vi "S&E Message Output.vi"(1 "All analog ch data":dbl[](array[numeric]), 2 "All digital Ch data":T2[](array[typedef]), 5 "Type(File Hist)":T1, 7 "E&S Message":T3, 9 "error in (no error)":errorcluster, 12 "Time format(%T)":string="%T", 13 "Delimiter(;)":string=";") -> (6 "String(File)":string, 8 "Array of strings":string[](array[string]), 10 "error out":errorcluster)   [LabVIEW 2011]
uses:
  emi Lib/System 01/0 - General/S&E reporting/Private/_emi_ S&E Message.ctl
  emi Lib/System 01/0 - General/S&E reporting/Private/_emi_ S&E Message type.ctl
  Measurments Handling/Status Digitalish.ctl
  String outpyt type.ctl
  reate/S&E Analog Alarm type.ctl
  GUI/Status Indikator Helper.ctl
  reate/S&E Event Type.ctl
  reate/S&E Event source.ctl
  reate/S&E Digital Alarm Type.ctl
  reate/S&E Anotationtype.ctl
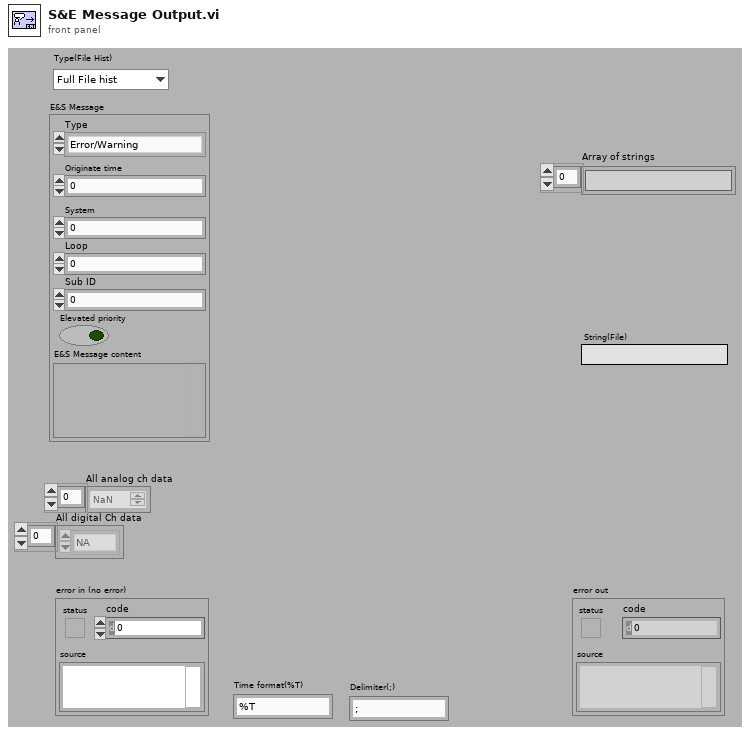
[diagram p1: front panel]
types:
  T1 = typedef "String outpyt type.ctl" = enum16{"Full File hist", "Simple File hist", "Displ Hist one type", "Displ Hist mult types", "Displ Stat one type", "Displ Stat Mult type"}
  T2 = typedef "Status Digitalish.ctl" = enum16{"NA", "False", "True"}
  T3 = typedef "_emi_ S&E Message.ctl" = cluster{"Type":T4, "Originate time":dbl, "System":u8, "Loop":u16, "Sub ID":u16, "Elevated priority":bool, "E&S Message content":variant}
  T4 = typedef "_emi_ S&E Message type.ctl" = enum16{"Error/Warning", "Note", "Debug", "Event", "Alarm Analog", "Alarm Digital", "Annotation"}
  T5 = typedef "S&E Analog Alarm type.ctl" = cluster{"Alarm":bool, "State":T6, "Value":dbl, "Source name":string}
  T6 = typedef "Status Indikator Helper.ctl" = enum16{"Norm", "L", "H", "LL", "HH", "Value", "Technical"}
  T7 = typedef "S&E Event Type.ctl" = cluster{"Event Source":T8, "Source Info":string, "Event Description":string}
  T8 = typedef "S&E Event source.ctl" = enum16{"User", "Instrument", "Application", "Windows"}
  T9 = typedef "S&E Digital Alarm Type.ctl" = cluster{"Alarm":bool, "Enum":T6, "Value":T2, "Source name":string, "Status text":string}
  T10 = typedef "S&E Anotationtype.ctl" = cluster{"User":string, "Annotation":string}
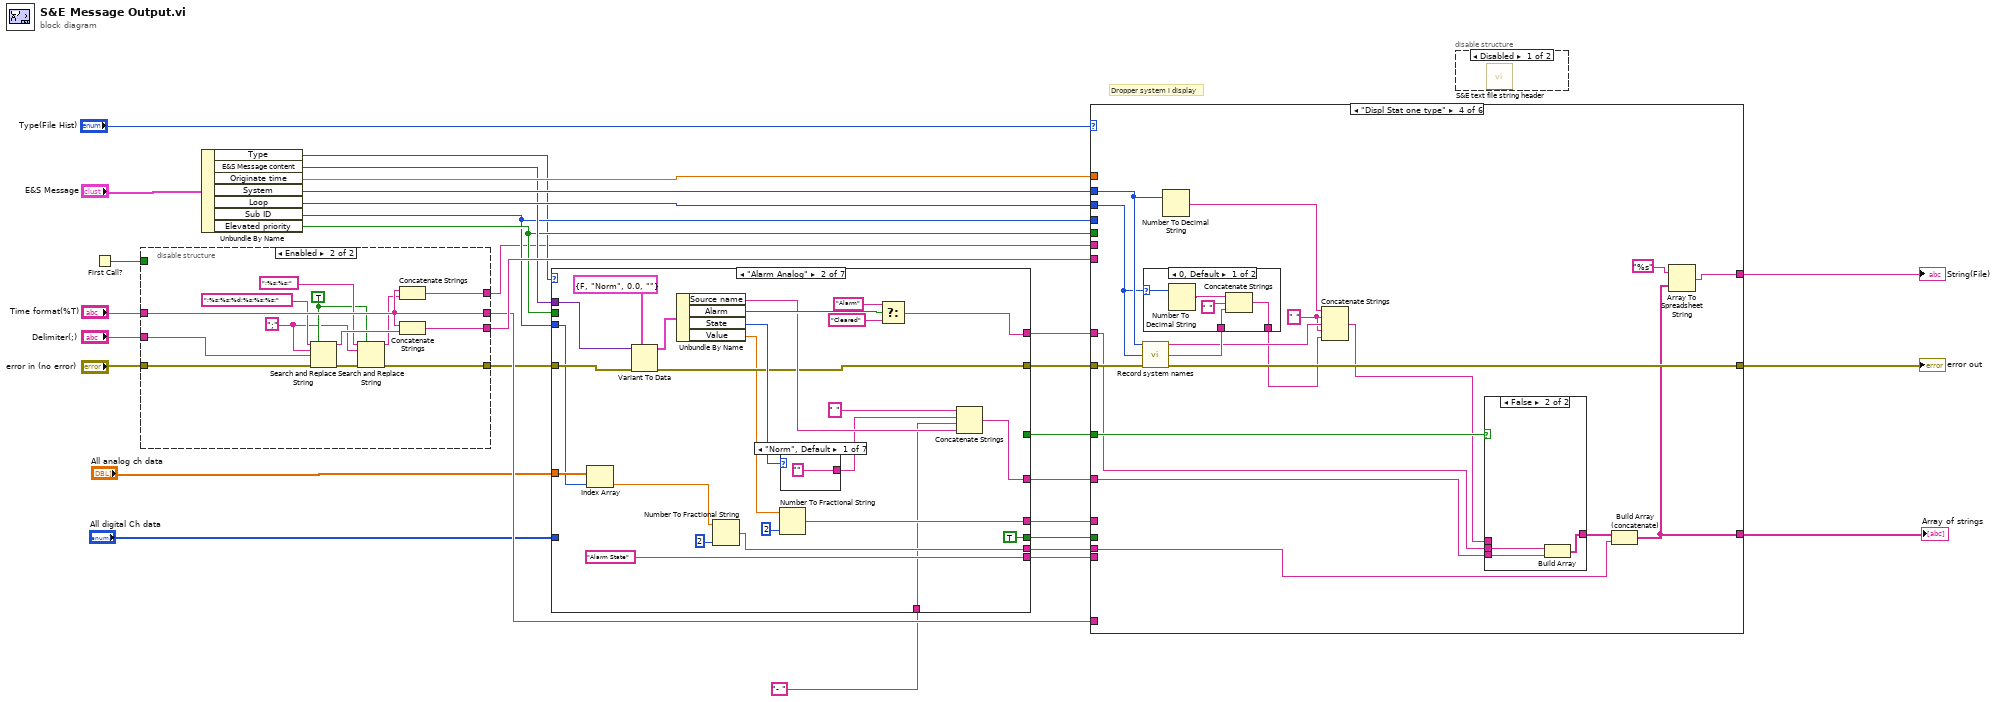
[diagram p0: block diagram]
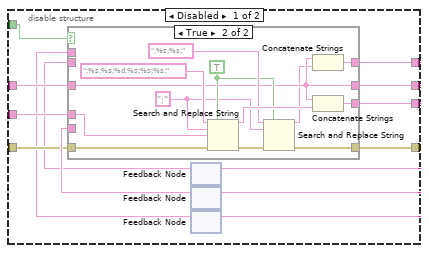
[diagram p2: hidden frame]
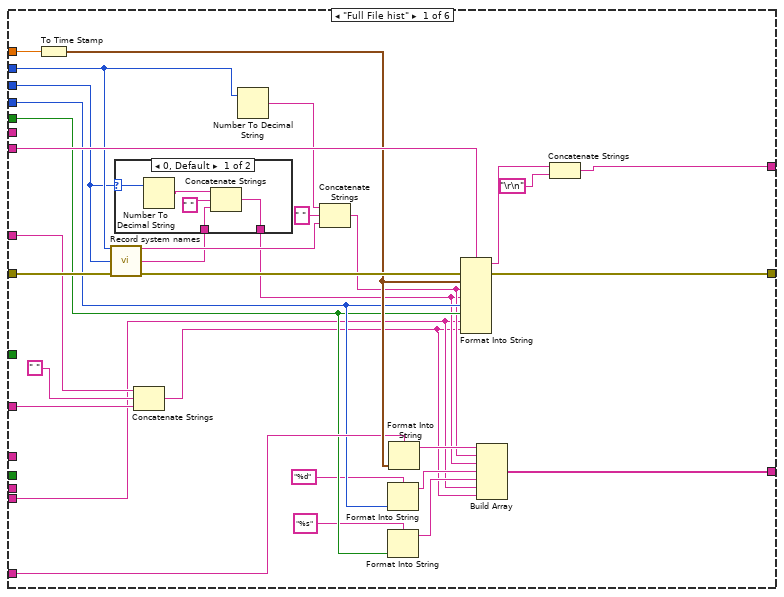
[diagram p5: hidden frame]
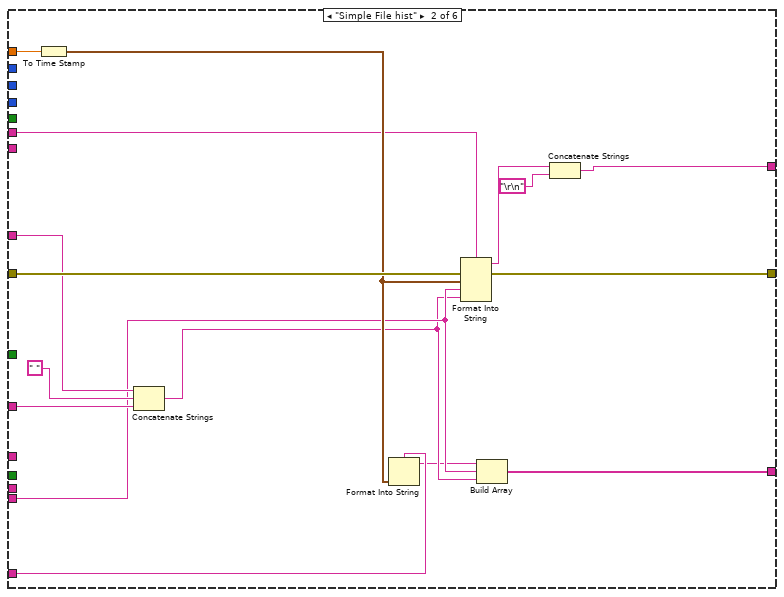
[diagram p7: hidden frame]
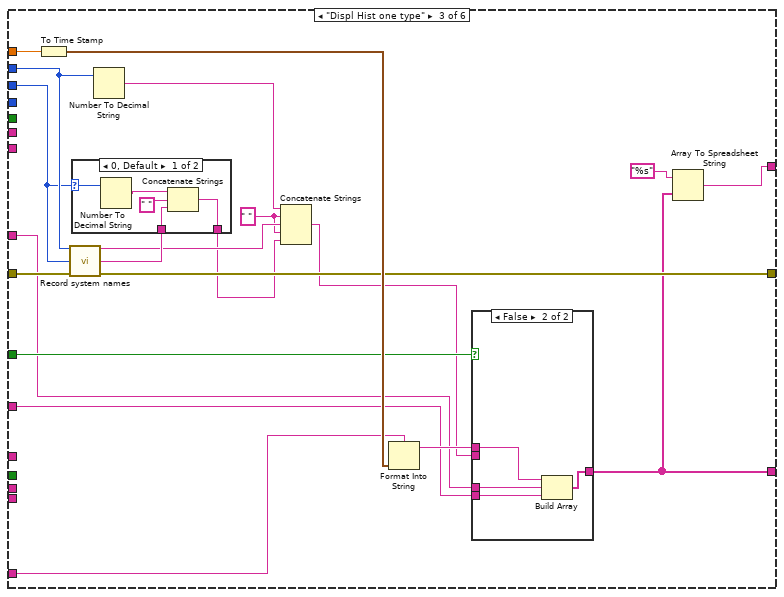
[diagram p8: hidden frame]
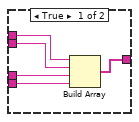
[diagram p9: hidden frame]
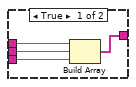
[diagram p11: hidden frame]
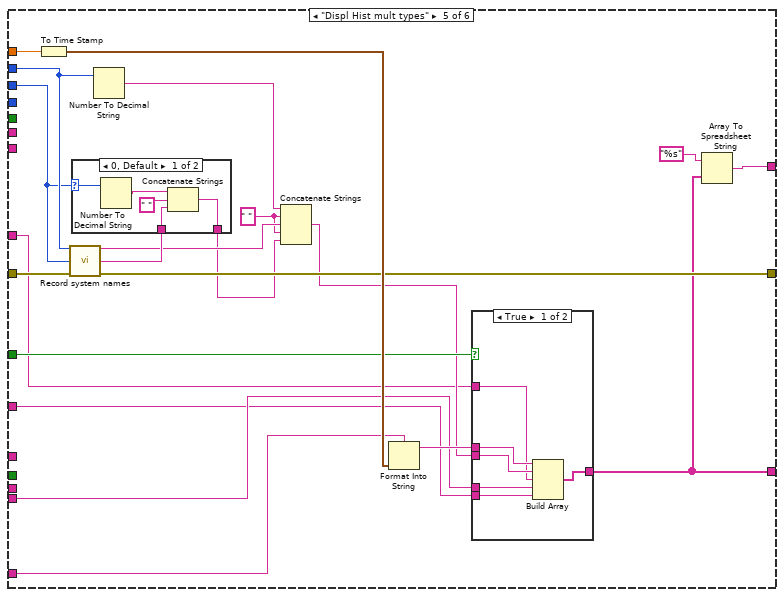
[diagram p13: hidden frame]
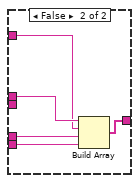
[diagram p14: hidden frame]
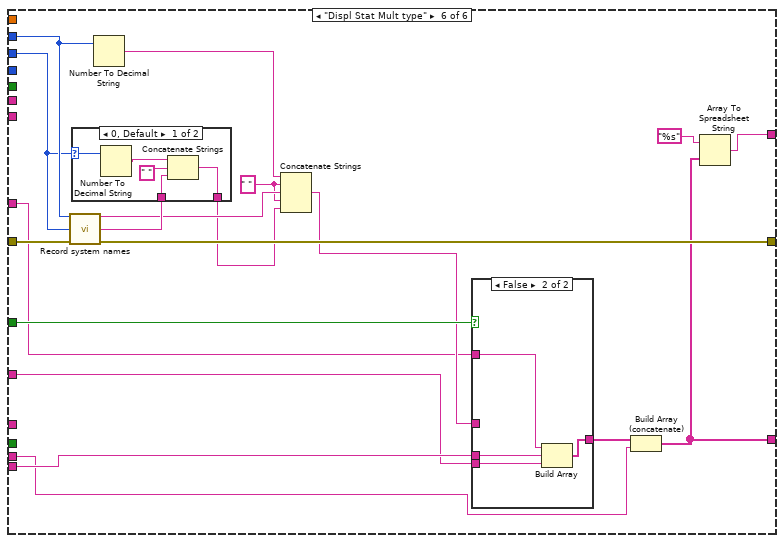
[diagram p16: hidden frame]
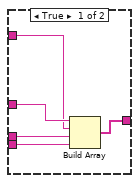
[diagram p17: hidden frame]
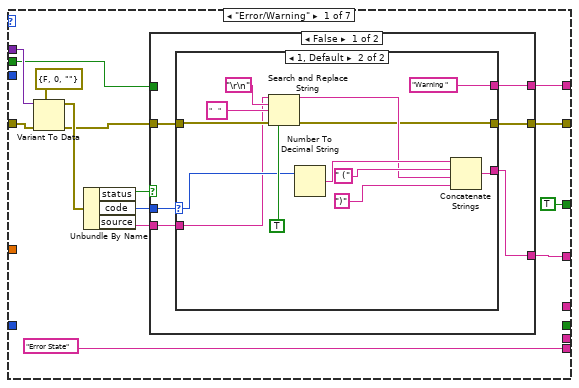
[diagram p19: hidden frame]
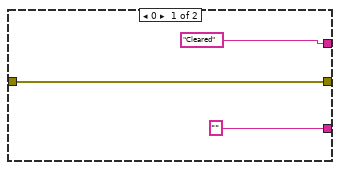
[diagram p20: hidden frame]
diagram:
  # "Dropper system i display"
  n1 = First Call?() -> (First Call?: T/F=w31:bool)
  n2 = disable-structure shown="Enabled" {
    disable-tunnel: w31 -> [w41 _]
    disable-tunnel: "Delimiter(;)" -> [w40 w72]
    disable-tunnel: "Time format(%T)" -> [w39 w69]
    disable-tunnel: "error in (no error)" -> [w38 w71]
    disable-tunnel: [w37 w70] -> w23
    disable-tunnel: [w35 w69] -> w20
    disable-tunnel: [w34 w68] -> w18
    disable-tunnel: [w32 w67] -> w2
    frame Disabled {
      n3 = feedback #1() -> (w33:string)  [unwired: 1 in]
      n4 = feedback #2() -> (w42:string)  [unwired: 1 in]
      n5 = feedback #3() -> (w36:string)  [unwired: 1 in]
      n6 = case shown="True" w41 {
        tunnel: [w46 w59] -> w37
        tunnel: w39 -> [_ w49]
        tunnel: w40 -> [_ w56]
        tunnel: w42 -> [w46 _]
        tunnel: [w45 w53] -> w34
        tunnel: w38 -> [w45 w55]
        tunnel: [w44 w49] -> w35
        tunnel: w36 -> [w44 _]
        tunnel: [w43 w47] -> w32
        tunnel: w33 -> [w43 _]
        frame False {
        }
        frame True {
          w51 = TRUE ("replace all? (F)")
          w50 = ";" ("search string")
          n7 = Search and Replace String(replace all?=w51, input string=";%s;%s;%d;%s;%s;%s;" ("format string"), search string=w50, replace string=w56, error in=w55) -> (result string=w58:string, error out=w54:errorcluster)  [unwired: 3 in, 2 out]
          n8 = Search and Replace String(replace all?=w51, input string=";%s;%s;" ("format string"), search string=w50, error in=w54) -> (result string=w48:string, error out=w53:errorcluster)  [unwired: 4 in, 2 out]
          n9 = Concatenate Strings(w49, w48) -> (w47:string)
          n10 = Concatenate Strings(w49, w58) -> (w59:string)
        }
      }
      n11 = feedback-in #1(w32) -> ()
      n12 = feedback-in #2(w37) -> ()
      n13 = feedback-in #3(w35) -> ()
    }
    frame Enabled {
      w62 = TRUE ("replace all? (F)")
      w61 = ";" ("search string")
      n14 = Search and Replace String(replace all?=w62, input string=";%s;%s;%d;%s;%s;%s;" ("format string"), search string=w61, replace string=w72, error in=w71) -> (result string=w66:string, error out=w64:errorcluster)  [unwired: 3 in, 2 out]
      n15 = Search and Replace String(replace all?=w62, input string=";%s;%s;" ("format string"), search string=w61, error in=w64) -> (result string=w60:string, error out=w68:errorcluster)  [unwired: 4 in, 2 out]
      n16 = Concatenate Strings(w69, w60) -> (w67:string)
      n17 = Concatenate Strings(w69, w66) -> (w70:string)
    }
  }
  n18 = Unbundle By Name("E&S Message") -> ("Type"=w9:T4, "E&S Message content"=w17:variant, "Originate time"=w26:dbl, "System"=w22:u8, "Loop"=w21:u16, "Sub ID"=w13:u16, "Elevated priority"=w16:bool)
  n19 = case shown="\"Alarm Analog\"" w9 {
    tunnel: [w75 w132 w160 w184 w207 w214 w222] -> w19
    tunnel: w18 -> [w83 w143 w164 w194 w210 w218 w225]
    tunnel: w17 -> [w82 w142 w163 w193 w209 w217 w224]
    tunnel: w16 -> [w79 _ _ _ _ _ _]
    tunnel: ["Error State" ("Time format(%T)") "Alarm State" ("Time format(%T)") "Event" ("Time format(%T)") "Alarm State" ("Time format(%T)") "User annotation" ("Time format(%T)") "Info" ("Time format(%T)") "Debug Message" ("Time format(%T)")] -> w12
    tunnel: [w76 w137 w157 w188 w204 _ _] -> w10
    tunnel: [w74 w133 w161 w185 w206 w215 w223] -> w11
    tunnel: [_ w130 _ w172 _ _ _] -> w6
    tunnel: "All analog ch data" -> [_ w129 _ _ _ _ _]
    tunnel: "All digital Ch data" -> [_ _ _ w181 _ _ _]
    tunnel: w13 -> [_ w128 _ w183 _ _ _]
    tunnel: [_ w126 _ w177 _ _ _] -> w5
    tunnel: [TRUE _ _ _ _ TRUE TRUE] -> w4
    tunnel: [_ TRUE _ TRUE _ _ _] -> w3
    tunnel: "- " ("string") -> [_ w122 w154 w179 _ _ _]
    frame "Error/Warning" {
      n20 = Variant To Data(error in=w83, type=errorcluster {"status"=FALSE, "code"=0, "source"=""} ("error in (no error)"), Variant=w82) -> (data=w84:errorcluster, error out=w80:errorcluster)
      n21 = Unbundle By Name(w84) -> ("status"=w81:bool, "code"=w78:i32, "source"=w77:string)
      n22 = case shown="False" w81 {
        tunnel: w80 -> [w92 w113]
        tunnel: w79 -> [_ _]
        tunnel: w78 -> [w87 w117]
        tunnel: w77 -> [w88 w112]
        tunnel: [w90 "Error" ("format string")] -> w76
        tunnel: [w91 w111] -> w75
        tunnel: [w89 w109] -> w74
        frame False {
          n23 = case shown="1, Default" w87 {
            selector: w87 -> [_ w99]
            tunnel: ["" w97] -> w89
            tunnel: [w95 w100] -> w91
            tunnel: w92 -> [w95 w101]
            tunnel: w88 -> [_ w98]
            tunnel: ["Cleared" ("format string") "Warning " ("format string")] -> w90
            frame 0 {
            }
            frame 1, Default {
              n24 = Search and Replace String(replace all?=TRUE ("replace all? (F)"), input string=w98, search string="\r\n", replace string="   " ("format string"), error in=w101) -> (result string=w104:string, error out=w100:errorcluster)  [unwired: 3 in, 2 out]
              n25 = Number To Decimal String(number=w99) -> (decimal integer string=w108:string)  [unwired: 1 in]
              n26 = Concatenate Strings(w108, " (" ("string"), w104, ")" ("string")) -> (w97:string)
            }
          }
        }
        frame True {
          n27 = Number To Decimal String(number=w117) -> (decimal integer string=w121:string)  [unwired: 1 in]
          n28 = Search and Replace String(replace all?=TRUE ("replace all? (F)"), input string=w112, search string="\r\n", replace string="   " ("format string"), error in=w113) -> (result string=w110:string, error out=w111:errorcluster)  [unwired: 3 in, 2 out]
          n29 = Concatenate Strings(w121, " (" ("string"), w110, ")" ("string")) -> (w109:string)
        }
      }
    }
    frame "Alarm Analog" {
      n30 = Index Array(array=w129, index=w128) -> (element=w127:dbl)
      n31 = Variant To Data(error in=w143, type=T5 {"Alarm"=FALSE, "State"=enum."Norm", "Value"=0.0, "Source name"=""} ("S&E Alarm"), Variant=w142) -> (data=w145:T5, error out=w132:errorcluster)
      n32 = Unbundle By Name(w145) -> ("Source name"=w135:string, "Alarm"=w140:bool, "State"=w138:T6, "Value"=w131:dbl)
      n33 = Number To Fractional String(number=w127, precision (6)=i16 2) -> (F-format string=w126:string)  [unwired: 2 in]
      n34 = Number To Fractional String(number=w131, precision (6)=i16 2) -> (F-format string=w130:string)  [unwired: 2 in]
      n35 = case shown="\"Norm\", Default" w138 {
        tunnel: ["" ("string") "L" ("string") "H" ("string") "LL" ("string") "HH" ("string") "Tech" ("string") "Dig" ("string")] -> w134
        frame "Norm", Default {
        }
        frame "L" {
        }
        frame "H" {
        }
        frame "LL" {
        }
        frame "HH" {
        }
        frame "Technical" {
        }
        frame "Value" {
        }
      }
      n36 = Select(t="Alarm", s=w140, f="Cleared") -> (s? t:f=w137:string)
      n37 = Concatenate Strings(" " ("string"), w134, w122, w135) -> (w133:string)
    }
    frame "Event" {
      n38 = Variant To Data(error in=w164, type=T7 {"Event Source"=enum."User", "Source Info"="", "Event Description"=""} ("S&E Event"), Variant=w163) -> (data=w165:T7, error out=w160:errorcluster)
      n39 = Unbundle By Name(w165) -> ("Event Description"=w155:string, "Source Info"=w156:string, "Event Source"=w158:T8)
      n40 = case shown="\"Application\"" w158 {
        tunnel: ["User" ("string") "Win." ("string") "Inst." ("string") "App." ("string")] -> w157
        frame "User", Default {
        }
        frame "Windows" {
        }
        frame "Instrument" {
        }
        frame "Application" {
        }
      }
      n41 = Concatenate Strings(w156, " " ("string"), w155, w154) -> (w161:string)
    }
    frame "Alarm Digital" {
      n42 = Index Array(array=w181, index=w183) -> (element=w178:T2)
      n43 = Variant To Data(error in=w194, type=T9 {"Alarm"=FALSE, "Enum"=enum."Norm", "Value"=enum."NA", "Source name"="", "Status text"=""} ("S&E Alarm"), Variant=w193) -> (data=w195:T9, error out=w184:errorcluster)
      n44 = Format Into String(format string="%s", w178) -> (resulting string=w177:string)  [unwired: 2 in, 1 out]
      n45 = Unbundle By Name(w195) -> ("Source name"=w171:string, "Alarm"=w191:bool, "Enum"=w189:T6, "Value"=w174:T2, "Status text"=w173:string)
      n46 = case shown="\"L\"" w189 {
        tunnel: ["" ("string") "L" ("string") "H" ("string") "LL" ("string") "HH" ("string") "Tech" ("string") "Val" ("string")] -> w186
        frame "Norm", Default {
        }
        frame "L" {
        }
        frame "H" {
        }
        frame "LL" {
        }
        frame "HH" {
        }
        frame "Technical" {
        }
        frame "Value" {
        }
      }
      n47 = Format Into String(format string="%s(%s)", w174, w173) -> (resulting string=w172:string)  [unwired: 2 in, 1 out]
      n48 = Select(t="Alarm", s=w191, f="Cleared") -> (s? t:f=w188:string)
      n49 = Concatenate Strings(" " ("string"), w186, w179, w171) -> (w185:string)
    }
    frame "Annotation" {
      (unwired) "   " ("string")
      n50 = Variant To Data(error in=w210, type=T10 {"User"="", "Annotation"=""} ("S&E Alarm"), Variant=w209) -> (data=w211:T10, error out=w207:errorcluster)
      n51 = Unbundle By Name(w211) -> ("User"=w204:string, "Annotation"=w208:string)
      n52 = Concatenate Strings(w208) -> (w206:string)
    }
    frame "Note" {
      n53 = Variant To Data(error in=w218, type="" ("Measage Header string"), Variant=w217) -> (data=w215:string, error out=w214:errorcluster)
    }
    frame "Debug" {
      n54 = Variant To Data(error in=w225, type="" ("Measage Header string"), Variant=w224) -> (data=w223:string, error out=w222:errorcluster)
    }
  }
  n55 = case shown="\"Displ Stat one type\"" "Type(File Hist)" {
    tunnel: [w231 w270 w280 w317 w347 w387] -> w30
    tunnel: w26 -> [w256 w278 w299 _ w366 _]
    tunnel: [w255 w277 w289 w326 w355 w395] -> w24
    tunnel: w23 -> [w254 _ _ _ _ _]
    tunnel: w22 -> [w249 _ w297 w331 w364 w401]
    tunnel: w21 -> [w248 _ w296 w330 w363 w400]
    tunnel: w20 -> [w242 w272 w292 _ w359 _]
    tunnel: w19 -> [w246 w276 w294 w328 w361 w398]
    tunnel: w16 -> [w240 _ _ _ _ _]
    tunnel: w13 -> [w241 _ _ _ _ _]
    tunnel: w12 -> [w228 w266 _ _ w357 w397]
    tunnel: w11 -> [w245 w275 w290 w327 w356 w396]
    tunnel: w10 -> [w244 w274 w283 w320 w349 w389]
    tunnel: [w232 w271 w282 w316 w346 w385] -> w7
    tunnel: w6 -> [_ _ _ _ _ _]
    tunnel: w5 -> [_ _ _ w315 _ w384]
    tunnel: w4 -> [_ _ w288 w325 w354 w394]
    tunnel: w3 -> [_ _ _ _ _ _]
    tunnel: w2 -> [_ w267 _ _ _ _]
    frame "Full File hist" {
      n56 = To Time Stamp(1:w256) -> (0:w243:timestamp)
      n57 = call "Record system names.vi"("System(0)"=w249, "Loop(0)"=w248, "error in (no error)"=w246) -> ("System navn"=w250:string, "Loop name"=w247:string, "error out"=w251:errorcluster)  [unwired: 8 in, 2 out]
      n58 = case shown="0, Default" w248 {
        selector: w248 -> [w258 _]
        tunnel: [w260 w263] -> w235
        tunnel: w247 -> [w259 w263]
        frame 0, Default {
          n59 = Number To Decimal String(number=w258) -> (decimal integer string=w262:string)  [unwired: 1 in]
          n60 = Concatenate Strings(w262, " " ("string"), w259) -> (w260:string)
        }
        frame 9999 {
        }
      }
      n61 = Concatenate Strings(w244, " " ("string"), w245) -> (w227:string)
      n62 = Number To Decimal String(number=w249) -> (decimal integer string=w252:string)  [unwired: 1 in]
      n63 = Concatenate Strings(w252, " " ("string"), w250) -> (w236:string)
      n64 = Format Into String(format string="%d", w241) -> (resulting string=w234:string)  [unwired: 2 in, 1 out]
      n65 = Format Into String(format string="%s", w240) -> (resulting string=w233:string)  [unwired: 2 in, 1 out]
      n66 = Format Into String(format string=w242, w243) -> (resulting string=w237:string)  [unwired: 2 in, 1 out]
      n67 = Format Into String(format string=w254, error in=w251, w243, w236, w235, w241, w240, w228, w227) -> (resulting string=w257:string, error out=w255:errorcluster)  [unwired: 1 in]
      n68 = Build Array(w237, w236, w235, w234, w233, w228, w227) -> (w232:string[])
      n69 = Concatenate Strings(w257, "\r\n") -> (w231:string)
    }
    frame "Simple File hist" {
      n70 = To Time Stamp(1:w278) -> (0:w273:timestamp)
      n71 = Concatenate Strings(w274, " " ("string"), w275) -> (w265:string)
      n72 = Format Into String(format string=w272, w273) -> (resulting string=w264:string)  [unwired: 2 in, 1 out]
      n73 = Format Into String(format string=w267, error in=w276, w273, w266, w265) -> (resulting string=w279:string, error out=w277:errorcluster)  [unwired: 1 in]
      n74 = Build Array(w264, w266, w265) -> (w271:string[])
      n75 = Concatenate Strings(w279, "\r\n") -> (w270:string)
    }
    frame "Displ Hist one type" {
      w286 = " " ("string")
      n76 = To Time Stamp(1:w299) -> (0:w293:timestamp)
      n77 = call "Record system names.vi"("System(0)"=w297, "Loop(0)"=w296, "error in (no error)"=w294) -> ("System navn"=w287:string, "Loop name"=w295:string, "error out"=w289:errorcluster)  [unwired: 8 in, 2 out]
      n78 = case shown="0, Default" w296 {
        selector: w296 -> [w309 _]
        tunnel: [w311 w314] -> w285
        tunnel: w295 -> [w310 w314]
        frame 0, Default {
          n79 = Number To Decimal String(number=w309) -> (decimal integer string=w313:string)  [unwired: 1 in]
          n80 = Concatenate Strings(w313, " " ("string"), w310) -> (w311:string)
        }
        frame 9999 {
        }
      }
      n81 = Number To Decimal String(number=w297) -> (decimal integer string=w298:string)  [unwired: 1 in]
      n82 = Concatenate Strings(w298, w286, w287, w286, w285) -> (w284:string)
      n83 = Format Into String(format string=w292, w293) -> (resulting string=w291:string)  [unwired: 2 in, 1 out]
      n84 = case shown="False" w288 {
        tunnel: w291 -> [w304 w308]
        tunnel: w284 -> [w303 _]
        tunnel: w283 -> [w302 w307]
        tunnel: [w301 w306] -> w282
        tunnel: w290 -> [w300 w305]
        frame True {
          n85 = Build Array(w304, w303, w302, w300) -> (w301:string[])
        }
        frame False {
          n86 = Build Array(w308, w307, w305) -> (w306:string[])
        }
      }
      n87 = Array To Spreadsheet String(array=w282, 3:"%s" ("Format")) -> (spreadsheet string=w280:string)  [unwired: 1 in]
    }
    frame "Displ Stat one type" {
      w323 = " " ("string")
      n88 = call "Record system names.vi"("System(0)"=w331, "Loop(0)"=w330, "error in (no error)"=w328) -> ("System navn"=w324:string, "Loop name"=w329:string, "error out"=w326:errorcluster)  [unwired: 8 in, 2 out]
      n89 = case shown="0, Default" w330 {
        selector: w330 -> [w340 _]
        tunnel: [w342 w345] -> w322
        tunnel: w329 -> [w341 w345]
        frame 0, Default {
          n90 = Number To Decimal String(number=w340) -> (decimal integer string=w344:string)  [unwired: 1 in]
          n91 = Concatenate Strings(w344, " " ("string"), w341) -> (w342:string)
        }
        frame 9999 {
        }
      }
      n92 = Number To Decimal String(number=w331) -> (decimal integer string=w332:string)  [unwired: 1 in]
      n93 = Concatenate Strings(w332, w323, w324, w323, w322) -> (w321:string)
      n94 = case shown="False" w325 {
        tunnel: w321 -> [w336 _]
        tunnel: w320 -> [w335 w339]
        tunnel: [w334 w338] -> w318
        tunnel: w327 -> [w333 w337]
        frame True {
          n95 = Build Array(w336, w335, w333) -> (w334:string[])
        }
        frame False {
          n96 = Build Array(w339, w337) -> (w338:string[])
        }
      }
      n97 = Build Array (concatenate)(w318, w315) -> (w316:string[])
      n98 = Array To Spreadsheet String(array=w316, 3:"%s" ("Format")) -> (spreadsheet string=w317:string)  [unwired: 1 in]
    }
    frame "Displ Hist mult types" {
      w352 = " " ("string")
      n99 = To Time Stamp(1:w366) -> (0:w360:timestamp)
      n100 = call "Record system names.vi"("System(0)"=w364, "Loop(0)"=w363, "error in (no error)"=w361) -> ("System navn"=w353:string, "Loop name"=w362:string, "error out"=w355:errorcluster)  [unwired: 8 in, 2 out]
      n101 = case shown="0, Default" w363 {
        selector: w363 -> [w378 _]
        tunnel: [w380 w383] -> w351
        tunnel: w362 -> [w379 w383]
        frame 0, Default {
          n102 = Number To Decimal String(number=w378) -> (decimal integer string=w382:string)  [unwired: 1 in]
          n103 = Concatenate Strings(w382, " " ("string"), w379) -> (w380:string)
        }
        frame 9999 {
        }
      }
      n104 = Number To Decimal String(number=w364) -> (decimal integer string=w365:string)  [unwired: 1 in]
      n105 = Concatenate Strings(w365, w352, w353, w352, w351) -> (w350:string)
      n106 = Format Into String(format string=w359, w360) -> (resulting string=w358:string)  [unwired: 2 in, 1 out]
      n107 = case shown="True" w354 {
        tunnel: w358 -> [w372 w377]
        tunnel: w350 -> [w371 _]
        tunnel: w357 -> [w370 w376]
        tunnel: [w369 w375] -> w346
        tunnel: w356 -> [w368 w374]
        tunnel: w349 -> [w367 w373]
        frame True {
          n108 = Build Array(w372, w371, w367, w370, w368) -> (w369:string[])
        }
        frame False {
          n109 = Build Array(w377, w373, w376, w374) -> (w375:string[])
        }
      }
      n110 = Array To Spreadsheet String(array=w346, 3:"%s" ("Format")) -> (spreadsheet string=w347:string)  [unwired: 1 in]
    }
    frame "Displ Stat Mult type" {
      w392 = " " ("string")
      n111 = call "Record system names.vi"("System(0)"=w401, "Loop(0)"=w400, "error in (no error)"=w398) -> ("System navn"=w393:string, "Loop name"=w399:string, "error out"=w395:errorcluster)  [unwired: 8 in, 2 out]
      n112 = case shown="0, Default" w400 {
        selector: w400 -> [w412 _]
        tunnel: [w414 w417] -> w391
        tunnel: w399 -> [w413 w417]
        frame 0, Default {
          n113 = Number To Decimal String(number=w412) -> (decimal integer string=w416:string)  [unwired: 1 in]
          n114 = Concatenate Strings(w416, " " ("string"), w413) -> (w414:string)
        }
        frame 9999 {
        }
      }
      n115 = Number To Decimal String(number=w401) -> (decimal integer string=w402:string)  [unwired: 1 in]
      n116 = Concatenate Strings(w402, w392, w393, w392, w391) -> (w390:string)
      n117 = case shown="False" w394 {
        tunnel: w390 -> [w407 _]
        tunnel: w397 -> [w406 w411]
        tunnel: [w405 w410] -> w386
        tunnel: w396 -> [w404 w409]
        tunnel: w389 -> [w403 w408]
        frame True {
          n118 = Build Array(w407, w403, w406, w404) -> (w405:string[])
        }
        frame False {
          n119 = Build Array(w408, w411, w409) -> (w410:string[])
        }
      }
      n120 = Build Array (concatenate)(w386, w384) -> (w385:string[])
      n121 = Array To Spreadsheet String(array=w385, 3:"%s" ("Format")) -> (spreadsheet string=w387:string)  [unwired: 1 in]
    }
  }
  "String(File)" <- w30
  "error out" <- w24
  "Array of strings" <- w7
  n122 = disable-structure shown="Disabled" {
    frame Disabled {
      n123 = call "S&E text file string header.vi"() -> ()  [unwired: 13 in, 3 out]
    }
    frame Enabled {
    }
  }
